vi "3 Tap 16-Bit.vi"() -> (0 "Pixels":T1)   [LabVIEW 2015]
uses:
  <vilib>/eio/EIONode/EIONode.xnode
  <vilib>/rvi/eio/common/nirviEmuTemplateMethod_errors.vi
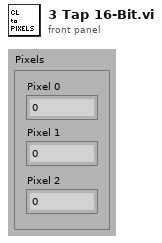
[diagram p1: front panel]
types:
  T1 = cluster{"Pixel 0":u16, "Pixel 1":u16, "Pixel 2":u16}
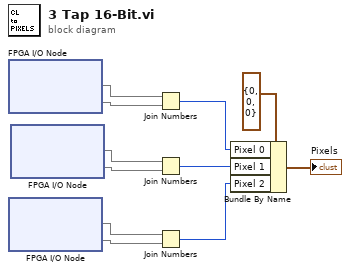
[diagram p0: block diagram]
diagram:
  n1 = xnode "FPGA I/O Node"() -> ("CL Port B"=w3, "CL Port A"=w9)  [unwired: 2 in, 2 out]
  n2 = xnode "FPGA I/O Node"() -> ("CL Port F"=w1, "CL Port C"=w8)  [unwired: 2 in, 2 out]
  n3 = xnode "FPGA I/O Node"() -> ("CL Port E"=w2, "CL Port D"=w7)  [unwired: 2 in, 2 out]
  n4 = Join Numbers(hi=w3, lo=w9) -> ((hi.lo)=w6:u32)
  n5 = Join Numbers(hi=w2, lo=w7) -> ((hi.lo)=w5:u32)
  n6 = Join Numbers(hi=w1, lo=w8) -> ((hi.lo)=w4:u32)
  n7 = Bundle By Name(cluster=T1 {"Pixel 0"=0, "Pixel 1"=0, "Pixel 2"=0} ("PixelData"), "Pixel 0"=w6, "Pixel 1"=w5, "Pixel 2"=w4) -> (→"Pixels":T1)
